vi "Configure Scan Measure.vi"(0 "VISA resource name":refnum<visa-resource-name>, 1 "Scan Count (0)":u32, 2 "Enable Route Bypass (T: Enable)":bool=TRUE, 5 "Event ID (\"NONE\")":string="NONE", 7 "Enable Scan Reset (T: Enable)":bool=TRUE, 9 "Channel List(\"\")":string, 11 "error in (no error)":errorcluster, 12 "Reading Buffer (\"\")":string, 13 "Interval (0 s)":dbl) -> (4 "VISA resource name out":refnum<visa-resource-name>, 15 "error out":errorcluster)   [LabVIEW 2015, in "Keithley DMM6500 DAQ6500 Series.lvlib"]
doc: "Configures the scan measurement."
uses:
  <instrlib>/Keithley DMM6500 DAQ6500 Series/Keithley DMM6500 DAQ6500 Series.lvlib
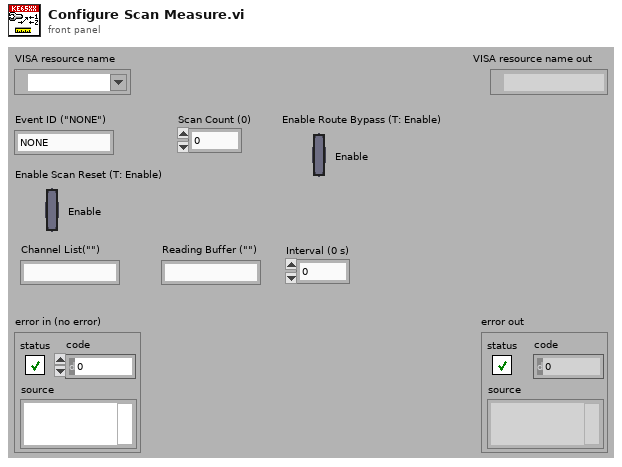
[diagram p1: front panel]
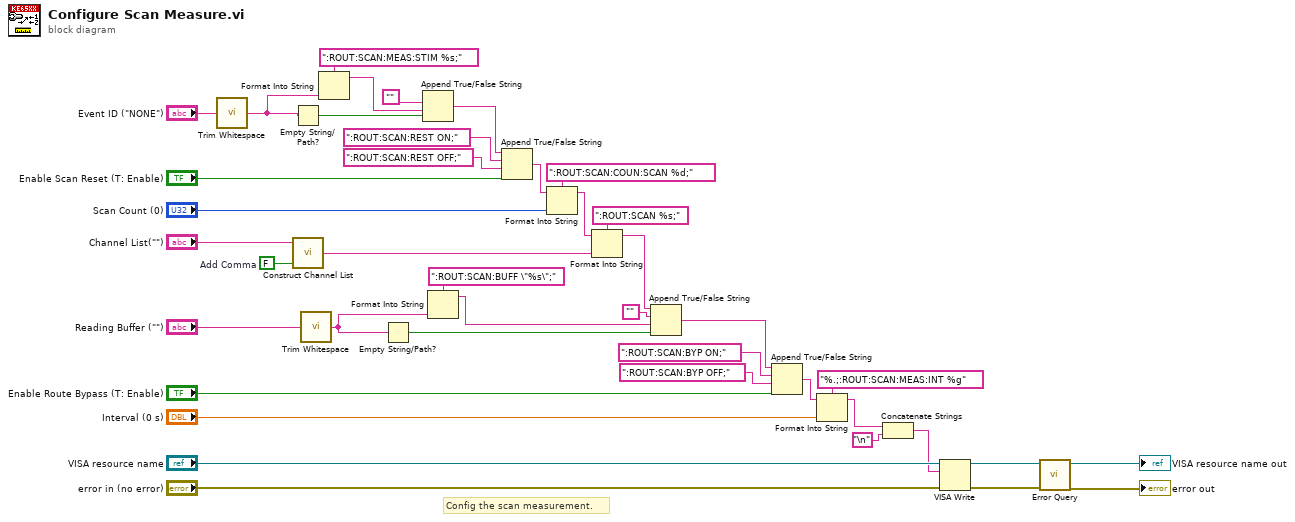
[diagram p0: block diagram]
diagram:
  w18 = FALSE  # Add Comma
  # "Config the scan measurement."
  n1 = call <vilib>:"Trim Whitespace.vi"("string"="Event ID (\"NONE\")") -> ("trimmed string"=w1:string)  [unwired: 1 in]
  n2 = Empty String/Path?(string/path=w1) -> (empty?=w2:bool)
  n3 = call <instrlib>:"Construct Channel List.vi"("Add Comma (True)"=w18, "Channel List"="Channel List(\"\")") -> ("Channel List String"=w19:string)  [unwired: 1 in]
  n4 = call <vilib>:"Trim Whitespace.vi"("string"="Reading Buffer (\"\")") -> ("trimmed string"=w3:string)  [unwired: 1 in]
  n5 = Format Into String(format string=":ROUT:SCAN:MEAS:STIM %s;", w1) -> (resulting string=w17:string)  [unwired: 2 in, 1 out]
  n6 = Empty String/Path?(string/path=w3) -> (empty?=w4:bool)
  n7 = Append True/False String(1:w2, 2:w17, 3:"") -> (0:w14:string)  [unwired: 1 in]
  n8 = Format Into String(format string=":ROUT:SCAN:BUFF \"%s\";", w3) -> (resulting string=w11:string)  [unwired: 2 in, 1 out]
  n9 = Append True/False String(1:"Enable Scan Reset (T: Enable)", 2:":ROUT:SCAN:REST OFF;", 3:":ROUT:SCAN:REST ON;", 4:w14) -> (0:w38:string)
  n10 = Format Into String(format string=":ROUT:SCAN:COUN:SCAN %d;", initial string=w38, "Scan Count (0)") -> (resulting string=w35:string)  [unwired: 1 in, 1 out]
  n11 = Format Into String(format string=":ROUT:SCAN %s;", initial string=w35, w19) -> (resulting string=w9:string)  [unwired: 1 in, 1 out]
  n12 = Append True/False String(1:w4, 2:w11, 3:"", 4:w9) -> (0:w8:string)
  n13 = Append True/False String(1:"Enable Route Bypass (T: Enable)", 2:":ROUT:SCAN:BYP OFF;", 3:":ROUT:SCAN:BYP ON;", 4:w8) -> (0:w29:string)
  n14 = Format Into String(format string="%.;:ROUT:SCAN:MEAS:INT %g", initial string=w29, "Interval (0 s)") -> (resulting string=w6:string)  [unwired: 1 in, 1 out]
  n15 = Concatenate Strings(w6, "\n") -> (w7:string)
  n16 = VISA Write(VISA resource name="VISA resource name", write buffer=w7, error in (no error)="error in (no error)") -> (VISA resource name out=w24:refnum<visa-resource-name>, error out=w23:errorcluster)  [unwired: 1 out]
  n17 = call <instrlib>:"Error Query.vi"("error in (no error)"=w23, "VISA resource name"=w24) -> ("error out"=→"error out":errorcluster, "VISA resource name out"=→"VISA resource name out":refnum<visa-resource-name>)  [unwired: 6 in, 2 out]
